vi "Format LogRecord.vi"(8 "error in":errorcluster, 10 "LogRecord":refnum<class "LogRecord.lvclass">, 11 "HSE_v2_Formatter in":refnum<class "HSE_v2_Formatter.lvclass">) -> (0 "error out":errorcluster, 2 "LogLine":string)   [LabVIEW 2024, in "hse-logger.lvlib" / "HSE_v2_Formatter.lvclass"]
doc: "Format the Log Record according the configured format string.\n\n____\nHAMPEL SOFTWARE ENGINEERING v2.2.2 (2025-01-16 15:41)"
uses:
  <vilib>/Hampel Software Engineering/HSE Logger/Formatter/HSE_v2_Formatter/HSE_v2_Formatter.lvclass
  C:/Program Files (x86)/National Instruments/LabVIEW 2024/vi.lib/Hampel Software Engineering/HSE Logger/Formatter/Formatter.lvclass
  <vilib>/Hampel Software Engineering/HSE Logger/LogRecord/LogRecord.lvclass
  <vilib>/Hampel Software Engineering/HSE Logger/Formatter/Formatter.lvclass/Formatter.ctl
  <vilib>/Hampel Software Engineering/HSE Logger/Formatter/HSE_v2_Formatter/HSE_v2_Formatter.lvclass/HSE_v2_Formatter.ctl
  <vilib>/Hampel Software Engineering/HSE Logger/LogRecord/LogRecord.lvclass/LogRecord.ctl
  <vilib>/Hampel Software Engineering/HSE Logger/Formatter/Formatter.lvclass
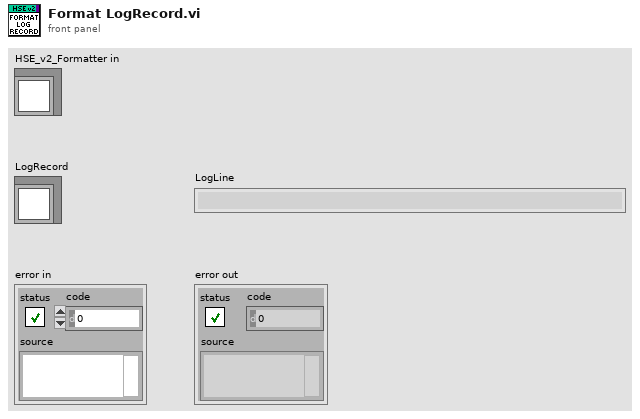
[diagram p1: front panel]
types:
  T1 = typedef "hse-logger.lvlib/LogLevel.ctl" = enum16{"DEBUG", "INFO", "WARNING", "ERROR", "CRITICAL"}
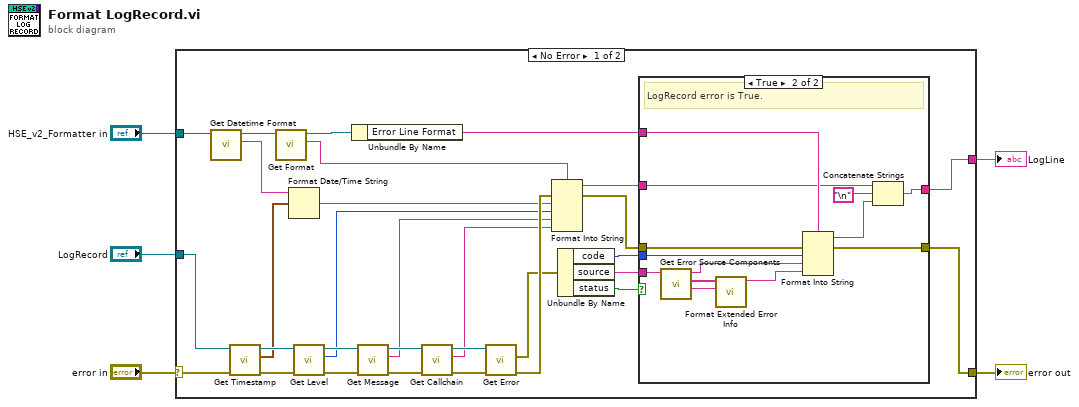
[diagram p0: block diagram]
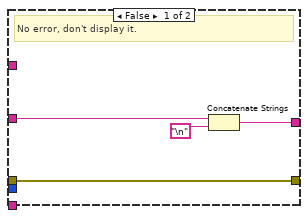
[diagram p2: hidden frame]
diagram:
  n1 = case shown="No Error" "error in" {
    selector: "error in" -> [w27 w53]
    tunnel: "HSE_v2_Formatter in" -> [w34 _]
    tunnel: "LogRecord" -> [w26 _]
    tunnel: [w7 _] -> w2
    tunnel: [w6 w53] -> w1
    frame No Error {
      n2 = call <vilib>:"Get Datetime Format.vi"("Formatter in"=w34) -> ("Datetime Format"=w21:string, "Formatter out"=w33:refnum<class "HSE_v2_Formatter.lvclass">)  [unwired: 8 in, 1 out]
      n3 = call <vilib>:"Get Timestamp.vi"("error in"=w27, "LogRecord in"=w26) -> ("error out"=w30:errorcluster, "Created"=w20:timestamp, "LogRecord out"=w25:refnum<class "LogRecord.lvclass">)  [unwired: 7 in]
      n4 = call <vilib>:"Get Format.vi"("Formatter in"=w33) -> ("Format"=w15:string, "Formatter out"=w32:refnum<class "HSE_v2_Formatter.lvclass">)  [unwired: 8 in, 1 out]
      n5 = Format Date/Time String(time format string (%c)=w21, seconds (now)=w20) -> (date/time string=w19:string)  [unwired: 1 in]
      n6 = call <vilib>:"Get Level.vi"("error in"=w30, "LogRecord in"=w25) -> ("error out"=w29:errorcluster, "Level"=w18:T1, "LogRecord out"=w24:refnum<class "LogRecord.lvclass">)  [unwired: 7 in]
      n7 = Unbundle By Name(w32) -> ("Error Line Format"=w14:string)
      n8 = call <vilib>:"Get Message.vi"("error in"=w29, "LogRecord in"=w24) -> ("error out"=w28:errorcluster, "Message"=w17:string, "LogRecord out"=w23:refnum<class "LogRecord.lvclass">)  [unwired: 7 in]
      n9 = call <vilib>:"Get Callchain.vi"("error in"=w28, "LogRecord in"=w23) -> ("error out"=w31:errorcluster, "Callchain"=w16:string, "LogRecord out"=w22:refnum<class "LogRecord.lvclass">)  [unwired: 7 in]
      n10 = call <vilib>:"Get Error.vi"("error in"=w31, "LogRecord in"=w22) -> ("error out"=w35:errorcluster, "Error"=w13:errorcluster)  [unwired: 7 in, 1 out]
      n11 = Format Into String(format string=w15, error in=w35, w19, w18, w17, w16) -> (resulting string=w9:string, error out=w8:errorcluster)  [unwired: 1 in]
      n12 = Unbundle By Name(w13) -> ("code"=w11:i32, "source"=w10:string, "status"=w12:bool)
      n13 = case shown="True" w12 {
        tunnel: w14 -> [_ w52]
        tunnel: w11 -> [_ w51]
        tunnel: w10 -> [_ w45]
        tunnel: w9 -> [w39 w49]
        tunnel: w8 -> [w37 w50]
        tunnel: [w38 w47] -> w7
        tunnel: [w37 w46] -> w6
        frame False {
          # "No error, don't display it."
          n14 = Concatenate Strings(w39, "\n") -> (w38:string)
        }
        frame True {
          # "LogRecord error is True."
          n15 = call <vilib>:"Get Error Source Components.vi"("Error Source String"=w45) -> ("DQMH Error Hint"=w41:string, "Call Chain"=w42:string[], "Error Message"=w43:string)  [unwired: 8 in]
          n16 = call <vilib>:"Format Extended Error Info.vi"("DQMH Error Hint"=w41, "Call Chain"=w42) -> ("Call Chain String"=w40:string)  [unwired: 9 in]
          n17 = Format Into String(format string=w52, error in=w50, w51, w43, w40) -> (resulting string=w48:string, error out=w46:errorcluster)  [unwired: 1 in]
          n18 = Concatenate Strings(w49, "\n", w48) -> (w47:string)
        }
      }
    }
    frame Error {
    }
  }
  "error out" <- w1
  "LogLine" <- w2
